vi "Module Identities.vi"(8 "error in (no error)":errorcluster, 11 "Log Manager Module in":refnum<class "Log Manager Module.lvclass">) -> (0 "error out":errorcluster, 2 "Identities":refnum<class "Identity.lvclass">[](array[class]), 3 "Log Manager Module out":refnum<class "Log Manager Module.lvclass">)   [LabVIEW 2020, in "VolatusData.lvlib" / "Log Manager Module.lvclass"]
uses:
  Log Manager Module.lvclass
  Volatus/Identity/Identity.lvclass
  Log Manager Module.lvclass/Log Manager Module.ctl
  Log Manager Identity/Log Manager Identity.lvclass
  C:/dev/lv20CE/relink/lv-volatus/VolatusData/Log Manager Identity/Log Manager Identity.lvclass
  C:/dev/lv20CE/relink/lv-volatus/Volatus/Identity/Identity.lvclass
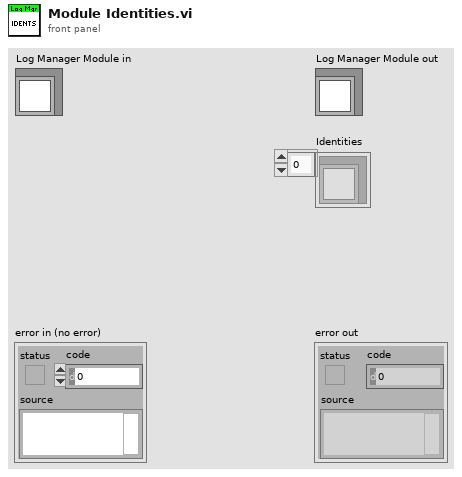
[diagram p1: front panel]
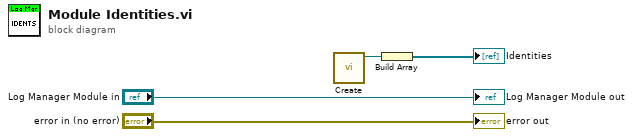
[diagram p0: block diagram]
diagram:
  n1 = call "Create.vi"() -> ("Log Manager Identity out"=w2:refnum<class "Log Manager Identity.lvclass">)  [unwired: 11 in]
  n2 = Build Array(w2) -> (→"Identities":refnum<class "Log Manager Identity.lvclass">[])
  "error out" <- "error in (no error)"
  "Log Manager Module out" <- "Log Manager Module in"
